vi "List Box Names.vi"(8 "error in (no error)":errorcluster, 11 "MulticolumnListbox in":refnum<vi>) -> (0 "error out":errorcluster, 2 "ItemNames":string[][](array[string]), 3 "MulticolumnListbox out":refnum<vi>)   [LabVIEW 2013, in "Table Manager.lvlib" / "Multi Column Listbox.lvclass"]
uses:
  Multi Column Listbox.lvclass
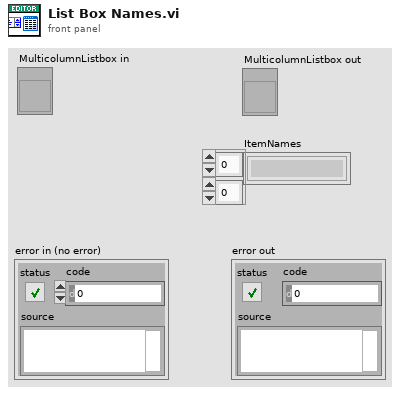
[diagram p1: front panel]
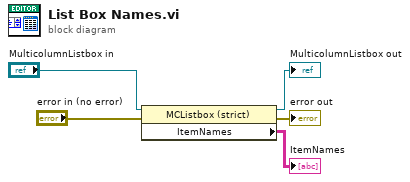
[diagram p0: block diagram]
diagram:
  n1 = property class="MCListbox (strict)"(reference="MulticolumnListbox in", error in="error in (no error)") -> (reference out=→"MulticolumnListbox out":refnum<vi>, error out=→"error out":errorcluster, "ItemNames"=→"ItemNames":string[][])
